vi "Multiple Straight Line Moves_safe.vi"() -> ()   [LabVIEW 2014]
doc: "This example shows a single axis straight-line move using the NI SoftMotion Line function block.\n\nNote: You must have the LabVIEW NI SoftMotion Module installed to run this example."
uses:
  <vilib>/Motion/Express/_s/nimc.fb.straightLineMove.startStraightLineMove.axis.modeRelative.0.vi
  <vilib>/Motion/Express/_s/nimc.fb.stopMove.stop.axis.modeDecelerate.vi
  <vilib>/Motion/Express/_s/nimc.fb.read.readExecutionData.axis.vi
  <vilib>/Motion/BlockNode/FB.NIMotion.xnode
panel:
  out "Acceleration (decimicrons/s2)":dbl
  out "Velocity (decimicrons/s)":dbl
  out "Position at Peak (decimicrons)":dbl
  in  "Target Peak Displacement (mm)":dbl
  in  "Target Pulse Duration (ms)":dbl
  out "Single Plot (Array of X,Y Pairs)":cluster{u32[], dbl[]}(graph)
  out "Example Done":bool=TRUE
  out "error out":errorcluster={"status"=FALSE, "code"=77003, "source"="Invoke Node in nimc.fb.straightLineMove.startStraightLineMove.axis.modeAbsolute.0.vi:5060005->Multiple Straight Line Moves.vi"}
  in  "Resource":refnum<k21>="Axis 1"
  # "Target Parameters"
  # "Computed Inputs"
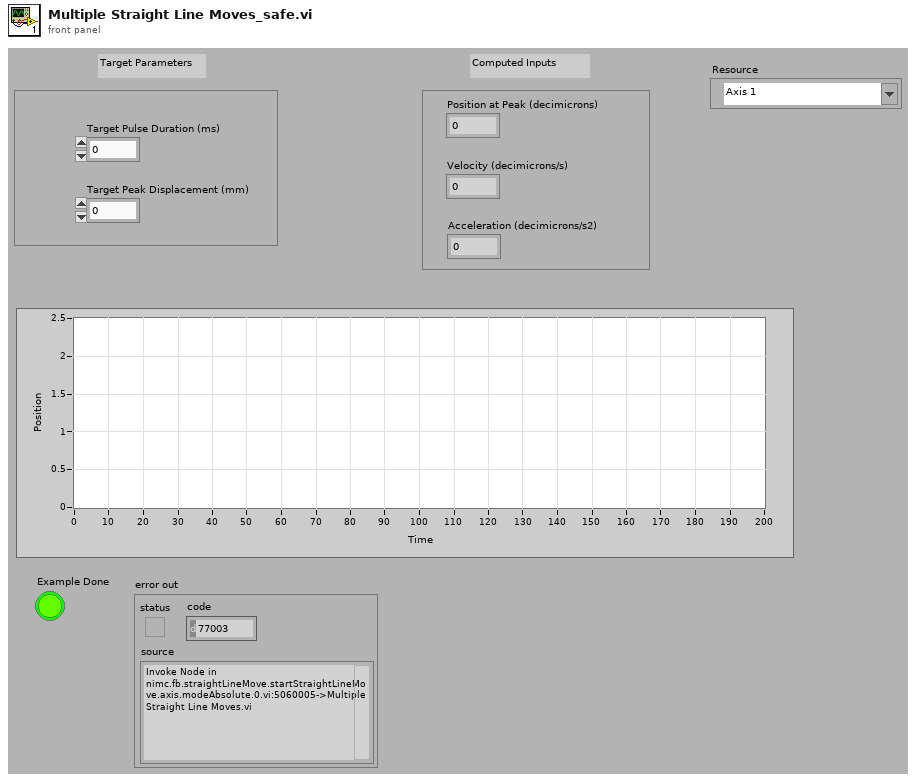
[diagram p1: front panel]
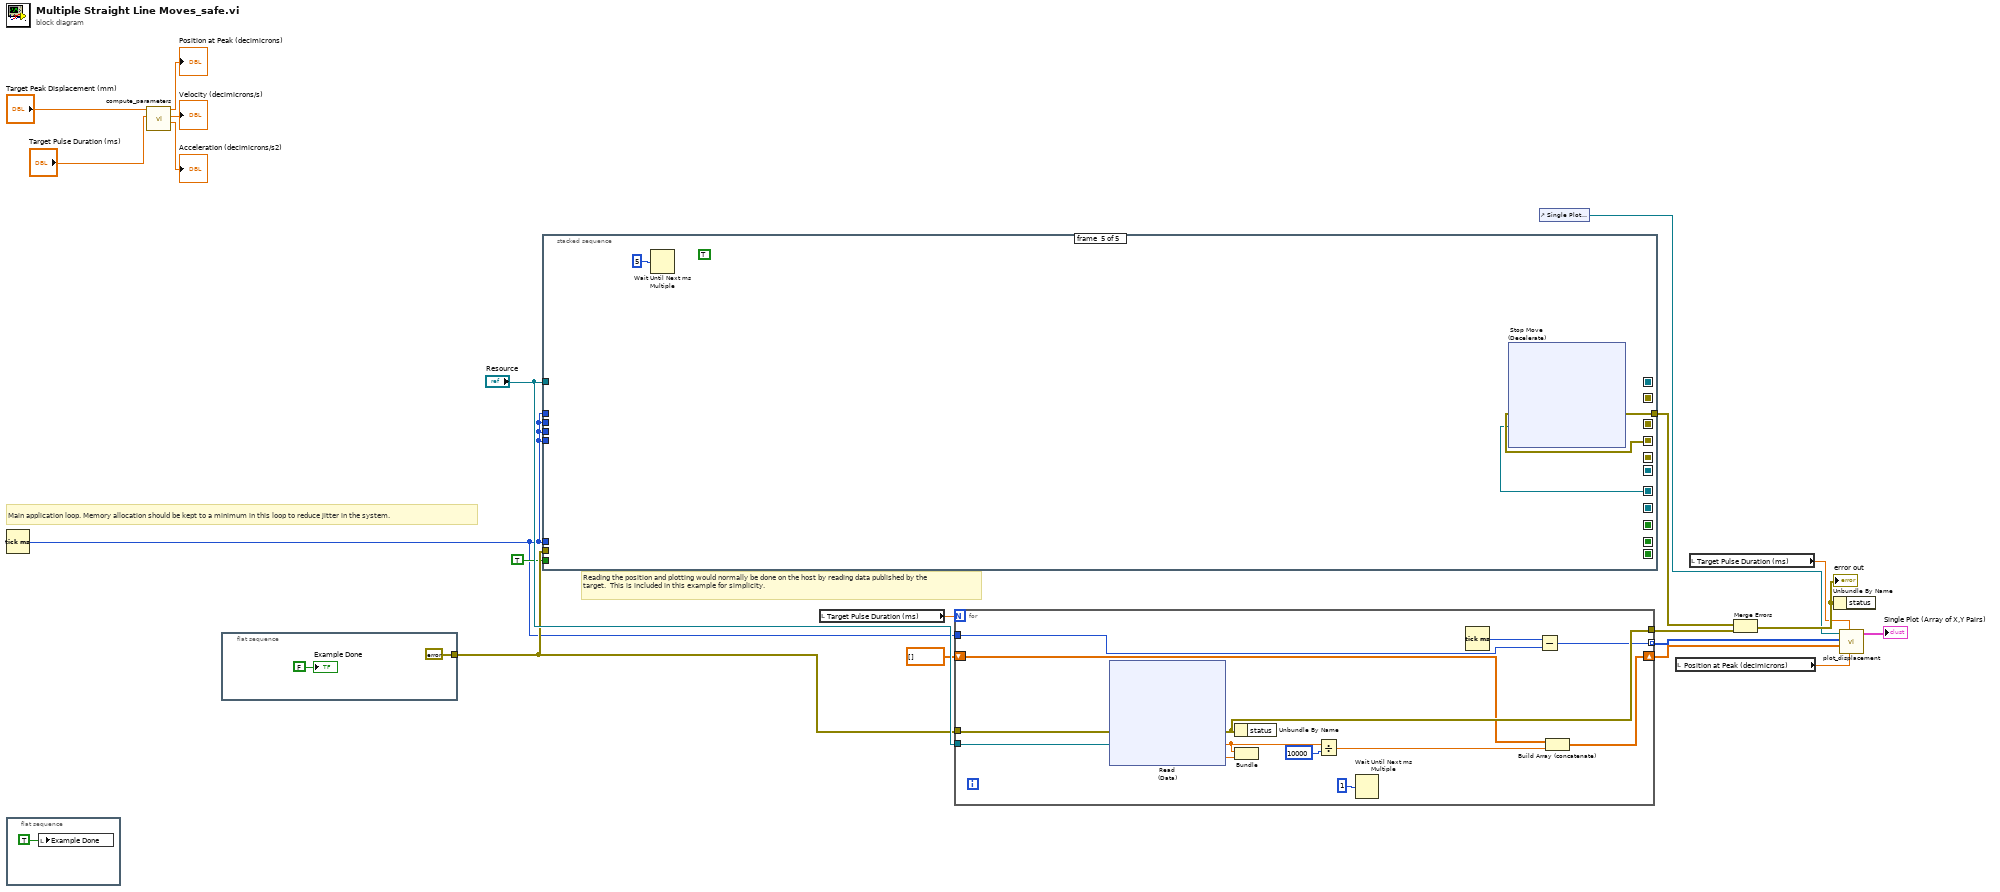
[diagram p0: block diagram]
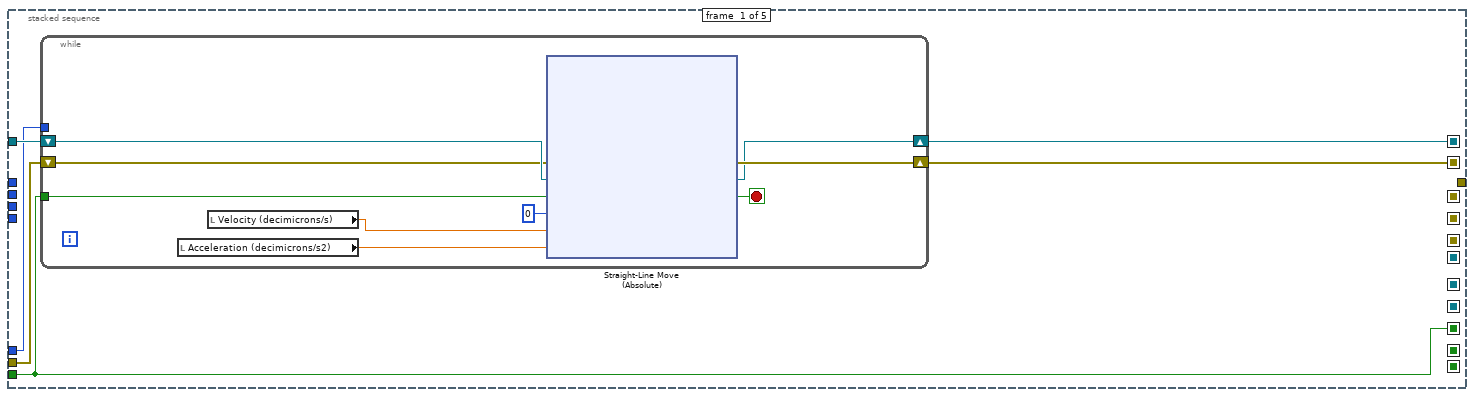
[diagram p2: hidden frame]
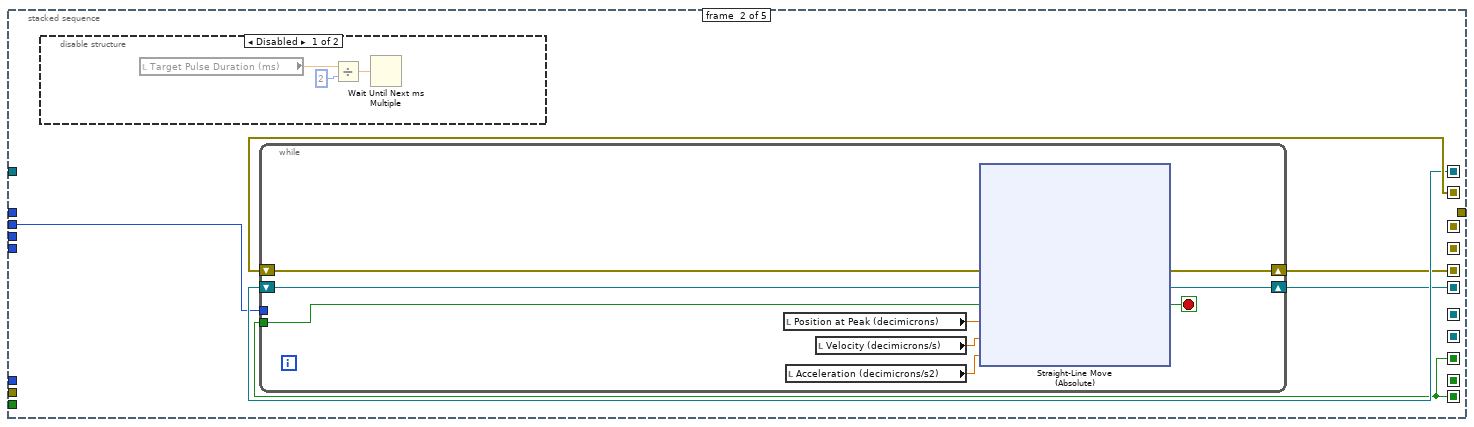
[diagram p3: hidden frame]
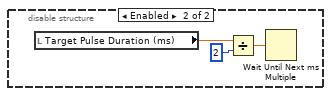
[diagram p4: hidden frame]
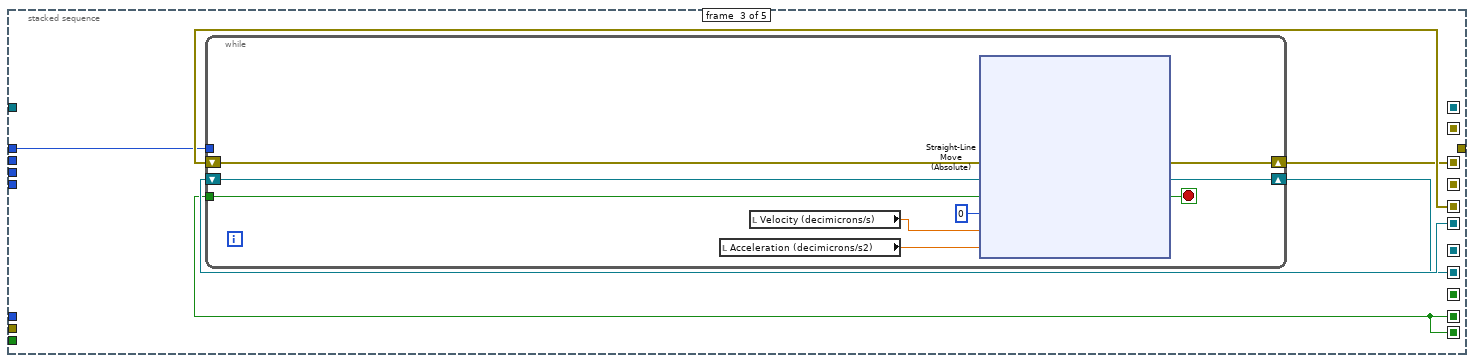
[diagram p5: hidden frame]
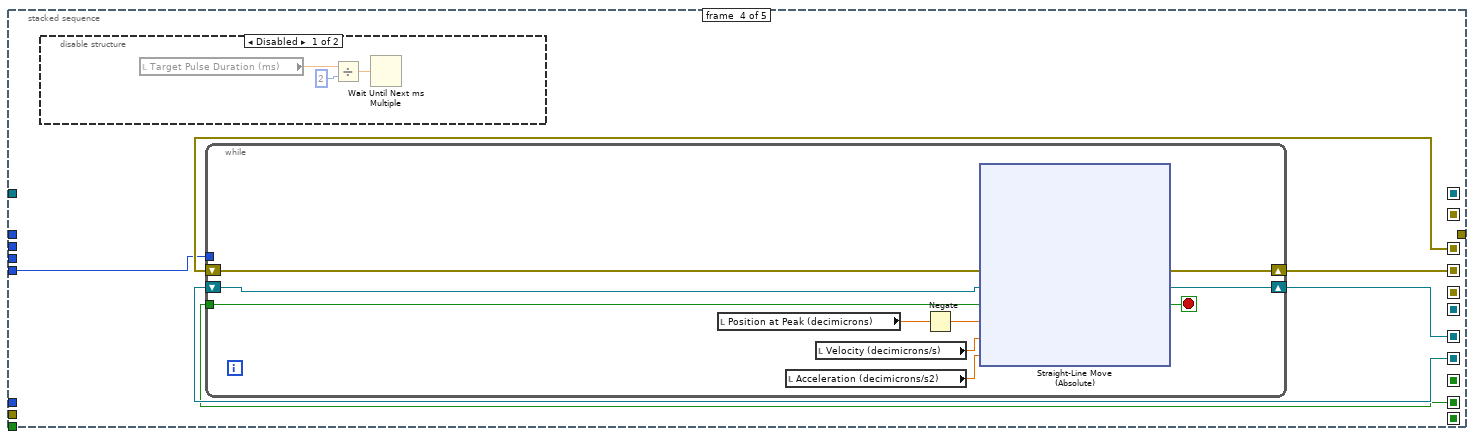
[diagram p6: hidden frame]
diagram:
  # "Reading the position and plotting would normally be done on the host by reading data published by the target.  This is included in this example for simplicity."
  # "Main application loop. Memory allocation should be kept to a minimum in this loop to reduce jitter in the system."
  n1 = Tick Count (ms)() -> (millisecond timer value=w14:u32)
  n2 = flat-sequence {
    frame #0 {
      n3 = local write "Example Done"(TRUE ("Example Done")) -> ()
    }
  }
  n4 = call "compute_parameters.vi"("Target Pulse Duration (ms)"="Target Pulse Duration (ms)", "Target Peak Displacement (mm)"="Target Peak Displacement (mm)") -> ("Numeric"=→"Acceleration (decimicrons/s2)":dbl, "Numeric 2"=→"Velocity (decimicrons/s)":dbl, "Position at Peak (decimicrons)"=→"Position at Peak (decimicrons)":dbl)  [unwired: 7 in]
  n5 = flat-sequence {
    tunnel: [errorcluster {"status"=FALSE, "code"=0, "source"=""} ("Error")] -> w19
    frame #0 {
      "Example Done" <- FALSE ("Example Done")
    }
  }
  n6 = stacked-sequence {
    seq-local: [w27 _ _ _ _] -> [_ w61 _ _ _]
    seq-local: [w26 _ _ _ _] -> [_ w60 _ _ _]
    seq-local: [w25 _ _ _ _] -> [_ w57 _ _ _]
    seq-local: [_ w59 _ _ _] -> [_ _ w99 _ _]
    seq-local: [_ w58 _ _ _] -> [_ _ w97 _ _]
    seq-local: [_ w57 _ _ _] -> [_ _ w95 _ _]
    seq-local: [_ _ w98 _ _] -> [_ _ _ w131 _]
    seq-local: [_ _ w96 _ _] -> [_ _ _ w129 _]
    seq-local: [_ _ w95 _ _] -> [_ _ _ w127 _]
    seq-local: [_ _ _ w130 _] -> [_ _ _ _ w165]
    seq-local: [_ _ _ w128 _] -> [_ _ _ _ w163]
    tunnel: "Resource" -> [w29 _ _ _ _]
    tunnel: w19 -> [w28 _ _ _ _]
    tunnel: TRUE ("approach forward") -> [w25 _ _ _ _]
    tunnel: w14 -> [w24 _ _ _ _]
    tunnel: w14 -> [_ w56 _ _ _]
    tunnel: w14 -> [_ _ w94 _ _]
    tunnel: w14 -> [_ _ _ w126 _]
    tunnel: [_ _ _ _ w164] -> w16
    tunnel: w14 -> [_ _ _ _ _]
    frame #0 {
      n7 = while {
        tunnel: w25 -> [w34]
        tunnel: w24 -> [_]
        shift-right: [w35] -> w26
        shift-left: w29 -> [w38]
        shift-right: [w36] -> w27
        shift-left: w28 -> [w37]
        stop <- w33 stop-if-true
        n8 = local read "Acceleration (decimicrons/s2)"() -> (w30:dbl)
        n9 = local read "Velocity (decimicrons/s)"() -> (w31:dbl)
        n10 = xnode "Straight-Line Move\n(Absolute)"("error in"=w37, "resource"=w38, "execute"=w34, "position"=0, "velocity"=w31, "acceleration"=w30) -> ("error out"=w36:errorcluster, "resource out"=w35:refnum<k21>, "done"=w33:bool)
      }
    }
    frame #1 {
      n11 = disable-structure shown="Disabled" {
        frame Disabled {
          n12 = local read "Target Pulse Duration (ms)"() -> (w64:dbl)
          n13 = Divide(x=w64, y=2) -> (x/y=w62:dbl)
          n14 = Wait Until Next ms Multiple(millisecond multiple=w62) -> ()  [unwired: 1 out]
        }
        frame Enabled {
          n15 = local read "Target Pulse Duration (ms)"() -> (w65:dbl)
          n16 = Divide(x=w65, y=2) -> (x/y=w66:dbl)
          n17 = Wait Until Next ms Multiple(millisecond multiple=w66) -> ()  [unwired: 1 out]
        }
      }
      n18 = while {
        tunnel: w57 -> [w72]
        tunnel: w56 -> [_]
        shift-right: [w74] -> w59
        shift-left: w61 -> [w76]
        shift-right: [w73] -> w58
        shift-left: w60 -> [w75]
        stop <- w68 stop-if-true
        n19 = local read "Position at Peak (decimicrons)"() -> (w71:dbl)
        n20 = local read "Acceleration (decimicrons/s2)"() -> (w69:dbl)
        n21 = local read "Velocity (decimicrons/s)"() -> (w70:dbl)
        n22 = xnode "Straight-Line Move\n(Absolute)"("error in"=w76, "resource"=w75, "execute"=w72, "position"=w71, "velocity"=w70, "acceleration"=w69) -> ("error out"=w74:errorcluster, "resource out"=w73:refnum<k21>, "done"=w68:bool)
      }
    }
    frame #2 {
      n23 = while {
        tunnel: w95 -> [w104]
        tunnel: w94 -> [_]
        shift-right: [w107] -> w98
        shift-left: w99 -> [w108]
        shift-right: [w105] -> w96
        shift-left: w97 -> [w106]
        stop <- w100 stop-if-true
        n24 = local read "Acceleration (decimicrons/s2)"() -> (w102:dbl)
        n25 = local read "Velocity (decimicrons/s)"() -> (w103:dbl)
        n26 = xnode "Straight-Line Move\n(Absolute)"("error in"=w108, "resource"=w106, "execute"=w104, "position"=0, "velocity"=w103, "acceleration"=w102) -> ("error out"=w107:errorcluster, "resource out"=w105:refnum<k21>, "done"=w100:bool)
      }
    }
    frame #3 {
      n27 = disable-structure shown="Disabled" {
        frame Disabled {
          n28 = local read "Target Pulse Duration (ms)"() -> (w132:dbl)
          n29 = Divide(x=w132, y=2) -> (x/y=w133:dbl)
          n30 = Wait Until Next ms Multiple(millisecond multiple=w133) -> ()  [unwired: 1 out]
        }
        frame Enabled {
        }
      }
      n31 = while {
        tunnel: w127 -> [w140]
        tunnel: w126 -> [_]
        shift-right: [w143] -> w130
        shift-left: w131 -> [w144]
        shift-right: [w141] -> w128
        shift-left: w129 -> [w142]
        stop <- w135 stop-if-true
        n32 = local read "Position at Peak (decimicrons)"() -> (w137:dbl)
        n33 = local read "Acceleration (decimicrons/s2)"() -> (w138:dbl)
        n34 = local read "Velocity (decimicrons/s)"() -> (w139:dbl)
        n35 = Negate(x=w137) -> (-x=w136:dbl)
        n36 = xnode "Straight-Line Move\n(Absolute)"("error in"=w144, "resource"=w142, "execute"=w140, "position"=w136, "velocity"=w139, "acceleration"=w138) -> ("error out"=w143:errorcluster, "resource out"=w141:refnum<k21>, "done"=w135:bool)
      }
    }
    frame #4 {
      (unwired) TRUE
      n37 = Wait Until Next ms Multiple(millisecond multiple=u32 5) -> ()  [unwired: 1 out]
      n38 = xnode "Stop Move\n(Decelerate)"("error in"=w165, "resource"=w163) -> ("error out"=w164:errorcluster)  [unwired: 1 in, 1 out]
    }
  }
  n39 = local read "Target Pulse Duration (ms)"() -> (w6:dbl)
  n40 = for {
    N: w6 -> [_]
    tunnel: "Resource" -> [w184]
    tunnel: w19 -> [w185]
    tunnel: [w182] -> w18
    tunnel: w14 -> [w180]
    shift-right: [w176] -> w4
    shift-left: dbl[] [] -> [w177]
    tunnel: [w173] -> w5 mode=indexing
    n41 = xnode "Read\n(Data)"("error in"=w185, "resource"=w184) -> ("error out"=w182:errorcluster, "position"=w178:dbl, "velocity"=w183:dbl)
    n42 = Unbundle By Name(w182) -> ()  [unwired: 1 out]
    n43 = Bundle("position"=w178, "velocity"=w183) -> ()  [unwired: 2 out]
    n44 = Divide(x=w178, y=10000) -> (x/y=w175:dbl)
    n45 = Wait Until Next ms Multiple(millisecond multiple=u32 1) -> ()  [unwired: 1 out]
    n46 = Tick Count (ms)() -> (millisecond timer value=w181:u32)
    n47 = Subtract(x=w181, y=w180) -> (x-y=w173:u32)
    n48 = Build Array (concatenate)(w177, w175) -> (w176:dbl[])
  }
  n49 = control-ref of="Single Plot (Array of X,Y Pairs)"() -> (w1:refnum<vi>)
  n50 = local read "Position at Peak (decimicrons)"() -> (w8:dbl)
  n51 = local read "Target Pulse Duration (ms)"() -> (w7:dbl)
  n52 = Merge Errors(w16, w18) -> (w15:errorcluster)
  "error out" <- w15
  n53 = Unbundle By Name(w15) -> ()  [unwired: 1 out]
  n54 = call "plot_displacement.vi"("Position at Peak (decimicrons)"=w8, "Target Pulse Duration (ms)"=w7, "Array"=w4, "Array 2"=w5, "XYGraph in"=w1) -> ("Cluster"=→"Single Plot (Array of X,Y Pairs)":cluster{u32[], dbl[]})  [unwired: 6 in]
